vi "CRYAPI Get Temp Reference.vi"(4 "Mode":bool, 5 "TitleName":string) -> (0 "TitleName Out":string, 1 "WindowType Out":string, 2 "VI Refnum":refnum<vi>)   [LabVIEW 2013]
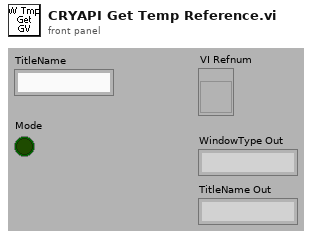
[diagram p1: front panel]
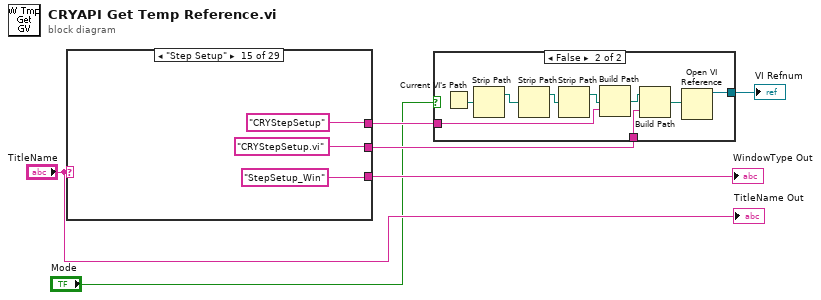
[diagram p0: block diagram]
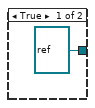
[diagram p2: hidden frame]
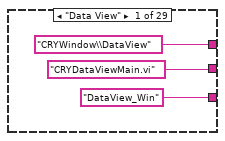
[diagram p3: hidden frame]
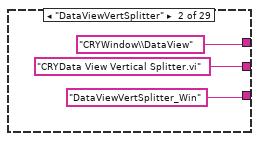
[diagram p4: hidden frame]
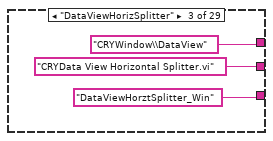
[diagram p5: hidden frame]
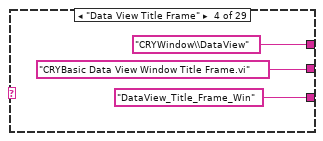
[diagram p6: hidden frame]
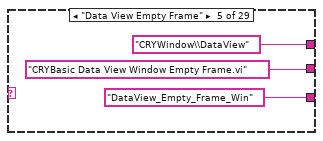
[diagram p7: hidden frame]
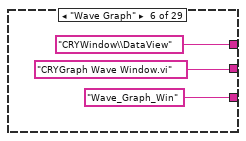
[diagram p8: hidden frame]
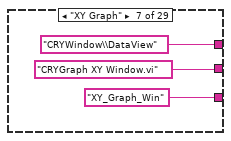
[diagram p9: hidden frame]
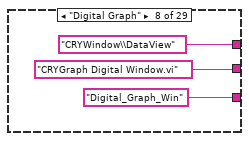
[diagram p10: hidden frame]
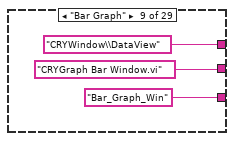
[diagram p11: hidden frame]
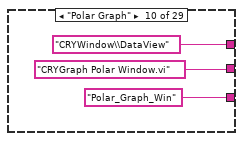
[diagram p12: hidden frame]
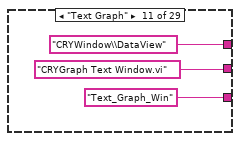
[diagram p13: hidden frame]
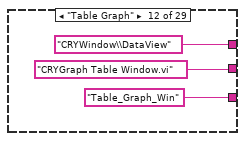
[diagram p14: hidden frame]
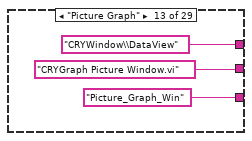
[diagram p15: hidden frame]
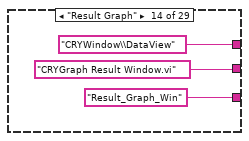
[diagram p16: hidden frame]
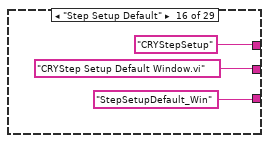
[diagram p17: hidden frame]
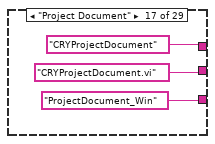
[diagram p18: hidden frame]
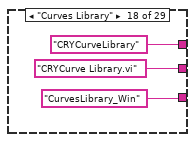
[diagram p19: hidden frame]
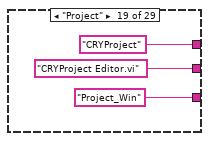
[diagram p20: hidden frame]
diagram:
  n1 = case shown="\"Step Setup\"" "TitleName" {
    tunnel: ["DataView_Win" ("Window Type 2") "DataViewVertSplitter_Win" ("Window Type 2") "DataViewHorztSplitter_Win" ("Window Type 2") "DataView_Title_Frame_Win" ("Window Type 2") "DataView_Empty_Frame_Win" ("Window Type 2") "Wave_Graph_Win" ("Window Type 2") "XY_Graph_Win" ("Window Type 2") "Digital_Graph_Win" ("Window Type 2") "Bar_Graph_Win" ("Window Type 2") "Polar_Graph_Win" ("Window Type 2") "Text_Graph_Win" ("Window Type 2") "Table_Graph_Win" ("Window Type 2") "Picture_Graph_Win" ("Window Type 2") "Result_Graph_Win" ("Window Type 2") "StepSetup_Win" ("Window Type 2") "StepSetupDefault_Win" ("Window Type 2") "ProjectDocument_Win" ("Window Type 2") "CurvesLibrary_Win" ("Window Type 2") "Project_Win" ("Window Type 2") "ResultView_Win" ("Window Type 2") "TAB_Win" ("Window Type 2") "AddStep_Win" ("Window Type 2") "AddStepTest1_Win" ("Window Type 2") "AddStepTest2_Win" ("Window Type 2") "MainVertSplitter_Win" ("Window Type 2") "MainHorizSplitter_Win" ("Window Type 2") "CenterEmpty_Win" ("Window Type 2") "BasicWindow_Win" ("Window Type 2") "Default_Win" ("Window Type 2")] -> w6
    tunnel: ["CRYWindow\\DataView" ("name") "CRYWindow\\DataView" ("name") "CRYWindow\\DataView" ("name") "CRYWindow\\DataView" ("name") "CRYWindow\\DataView" ("name") "CRYWindow\\DataView" ("name") "CRYWindow\\DataView" ("name") "CRYWindow\\DataView" ("name") "CRYWindow\\DataView" ("name") "CRYWindow\\DataView" ("name") "CRYWindow\\DataView" ("name") "CRYWindow\\DataView" ("name") "CRYWindow\\DataView" ("name") "CRYWindow\\DataView" ("name") "CRYStepSetup" ("name") "CRYStepSetup" ("name") "CRYProjectDocument" ("name") "CRYCurveLibrary" ("name") "CRYProject" ("name") "CRYResultView" ("name") "CRYWindow\\Tab" ("name") "CRYAddStep" ("name") "CRYAddStep" ("name") "CRYAddStep" ("name") "CRYWindow\\SubVI" ("name") "CRYWindow\\SubVI" ("name") "CRYWindow\\SubVI" ("name") "CRYWindow\\SubVI" ("name") "CRYWindow\\SubVI" ("name")] -> w4
    tunnel: ["CRYDataViewMain.vi" ("name") "CRYData View Vertical Splitter.vi" ("name") "CRYData View Horizontal Splitter.vi" ("name") "CRYBasic Data View Window Title Frame.vi" ("name") "CRYBasic Data View Window Empty Frame.vi" ("name") "CRYGraph Wave Window.vi" ("name") "CRYGraph XY Window.vi" ("name") "CRYGraph Digital Window.vi" ("name") "CRYGraph Bar Window.vi" ("name") "CRYGraph Polar Window.vi" ("name") "CRYGraph Text Window.vi" ("name") "CRYGraph Table Window.vi" ("name") "CRYGraph Picture Window.vi" ("name") "CRYGraph Result Window.vi" ("name") "CRYStepSetup.vi" ("name") "CRYStep Setup Default Window.vi" ("name") "CRYProjectDocument.vi" ("name") "CRYCurve Library.vi" ("name") "CRYProject Editor.vi" ("name") "CRYResult View Main.vi" ("name") "CRYTab Main.vi" ("name") "CRYAdd Steps.vi" ("name") "test_GVAdd Steps1.vi" ("name") "test_GVAdd Steps2.vi" ("name") "CRYMain Vertical Splitter.vi" ("name") "CRYMain Horizontal Splitter.vi" ("name") "CRYMain Center Empty.vi" ("name") "CRYBasic Window Frame.vi" ("name") "CRYDefault Window.vi" ("name")] -> w3
    frame "Data View" {
    }
    frame "DataViewVertSplitter" {
    }
    frame "DataViewHorizSplitter" {
    }
    frame "Data View Title Frame" {
    }
    frame "Data View Empty Frame" {
    }
    frame "Wave Graph" {
    }
    frame "XY Graph" {
    }
    frame "Digital Graph" {
    }
    frame "Bar Graph" {
    }
    frame "Polar Graph" {
    }
    frame "Text Graph" {
    }
    frame "Table Graph" {
    }
    frame "Picture Graph" {
    }
    frame "Result Graph" {
    }
    frame "Step Setup" {
    }
    frame "Step Setup Default" {
    }
    frame "Project Document" {
    }
    frame "Curves Library" {
    }
    frame "Project" {
    }
    frame "Result View" {
    }
    frame "TAB" {
    }
    frame "Add Step" {
    }
    frame "AddStepTest1" {
    }
    frame "AddStepTest2" {
    }
    frame "MainVertSplitter" {
    }
    frame "MainHorizSplitter" {
    }
    frame "CenterEmpty" {
    }
    frame "BasicWindow" {
    }
    frame "", Default {
    }
  }
  "WindowType Out" <- w6
  n2 = case shown="False" "Mode" {
    tunnel: w4 -> [_ w99]
    tunnel: w3 -> [_ w98]
    tunnel: [refnum<vi> refnum w97] -> w2
    frame True {
    }
    frame False {
      n3 = Current VI's Path() -> (path=w96:path)
      n4 = Strip Path(path=w96) -> (stripped path=w95:path)  [unwired: 1 out]
      n5 = Strip Path(path=w95) -> (stripped path=w100:path)  [unwired: 1 out]
      n6 = Strip Path(path=w100) -> (stripped path=w102:path)  [unwired: 1 out]
      n7 = Build Path(base path=w102, name or relative path=w99) -> (appended path=w101:path)
      n8 = Build Path(base path=w101, name or relative path=w98) -> (appended path=w103:path)
      n9 = Open VI Reference(vi path=w103) -> (vi reference=w97:refnum<vi>)  [unwired: 1 in, 5 out]
    }
  }
  "VI Refnum" <- w2
  "TitleName Out" <- "TitleName"
